vi "SetParam.vi"(8 "error in (no error)":errorcluster caption="entrée d'erreur (pas d'erreur)", 10 "rbf_kernel":cluster{"gamma":string}={"gamma"="None"}, 11 "Rbf_kernel.lvclass":refnum<class "Rbf_kernel.lvclass">) -> (0 "error out":errorcluster caption="sortie d'erreur", 3 "Rbf_kernel.lvclass":refnum<class "Rbf_kernel.lvclass">)   [LabVIEW 2020, in "Rbf_kernel.lvclass"]
doc: "Set Parameters"
uses:
  Rbf_kernel.lvclass
  Rbf_kernel.lvclass/Rbf_kernel.ctl
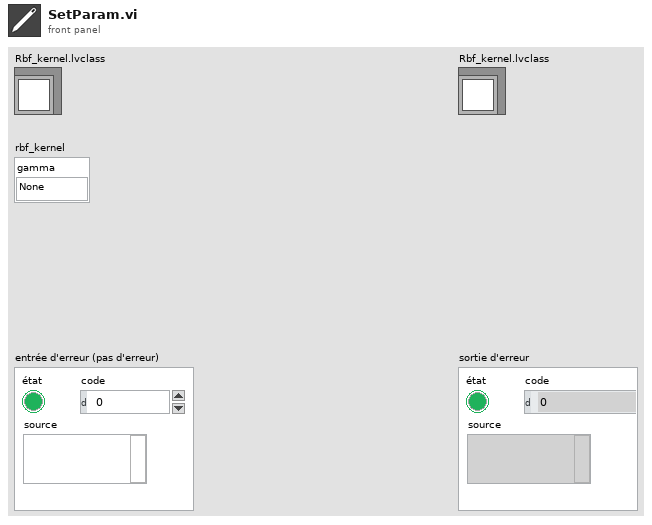
[diagram p1: front panel]
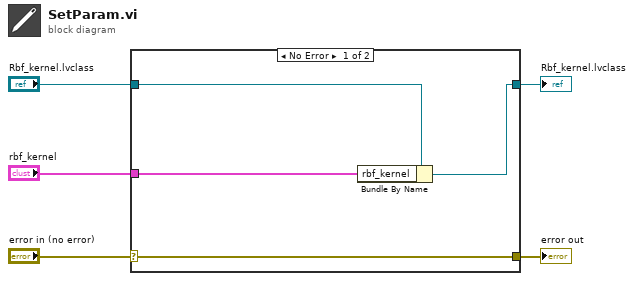
[diagram p0: block diagram]
diagram:
  n1 = case shown="No Error" "error in (no error)" {
    selector: "error in (no error)" -> [w9 w10]
    tunnel: [w9 w10] -> w4
    tunnel: [w7 w11] -> w2
    tunnel: "Rbf_kernel.lvclass" -> [w8 w11]
    tunnel: "rbf_kernel" -> [w6 _]
    frame No Error {
      n2 = Bundle By Name(cluster=w8, "rbf_kernel"=w6) -> (w7:refnum<class "Rbf_kernel.lvclass">)
    }
    frame Error {
    }
  }
  "error out" <- w4
  "Rbf_kernel.lvclass" <- w2
